vi "countrateJ&J.vi"() -> ()   [LabVIEW 2015]
uses:
  <vilib>/Platform/TimedLoop/XDataNode/timing_clust.ctl
  <vilib>/Platform/TimedLoop/XDataNode/nitl_modes.ctl
  <vilib>/Platform/TimedLoop/XDataNode/wakeup.ctl
  <vilib>/platform/TimedLoop/XDataNode/XDataNode.xnode
  <vilib>/Platform/TimedLoop/XDataNode/XDNodeRunTimeDep.lvlib
panel:
  out "Countrate":cluster{i32[], i32[]}(graph)
  out "output cluster":cluster{i32, dbl}
  in  "Controls":T1
  out "counts per Time Increment":dbl(knob) scale=0.0..100.0
  in  "stop":bool
  # "Demo count rate VI for Physics 434"
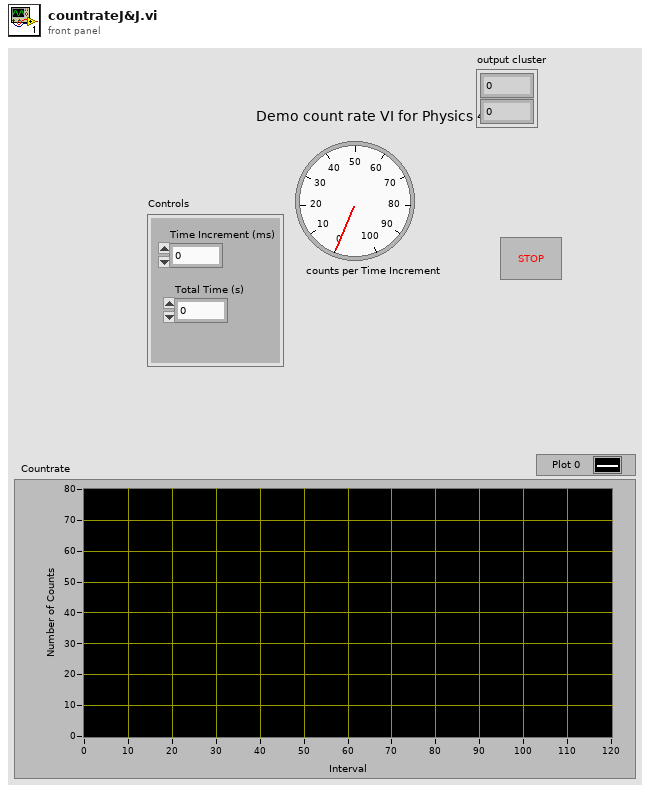
[diagram p1: front panel]
types:
  T1 = cluster{"Time Increment (ms)":i64, "Total Time (s)":dbl}
  T2 = enum16{"open", "replace", "create", "open or create", "replace or create", "replace or create with confirmation"}
  T3 = typedef "XDNodeRunTimeDep.lvlib/timing_clust.ctl" = cluster{"Expected End [f-1]":u64, "Actual End [f-1]":u64, "Finished Late? [f-1]":bool, "Expected End [i-1]":u64, "Actual End [i-1]":u64, "Finished Late? [i-1]":bool, "Expected Start [i]":u64, "Actual Start [i]":u64, "Expected Start [f]":u64, "Actual Start [f]":u64, "Source Name":string, "Structure Name":string, "Period":i64, "Deadline":i64, "Offset":i64, "Start":i64, "Priority":i32, "Timeout":i32, "Mode":T4, "Wakeup Reason":T5, "Error":errorcluster, "Source Type":string, "Secondary Source Type":string, "Global End Time":u64, "Global Start Time":u64, "Frame Duration":u64, "Iteration Duration":u64, "Assigned CPU":i32, "I/O Scan Engine Mode":u32}
  T4 = typedef "XDNodeRunTimeDep.lvlib/nitl_modes.ctl" = enum32{"No Change", "Process missed periods, maintain original phase", "Discard missed periods, maintain original phase", "Process missed periods, ignore original phase", "Discard missed periods, ignore original phase"}
  T5 = typedef "XDNodeRunTimeDep.lvlib/wakeup.ctl" = enum32{"Normal", "Aborted", "Asynchronous wakeup", "Timing source error", "Timed loop error", "Timeout"}
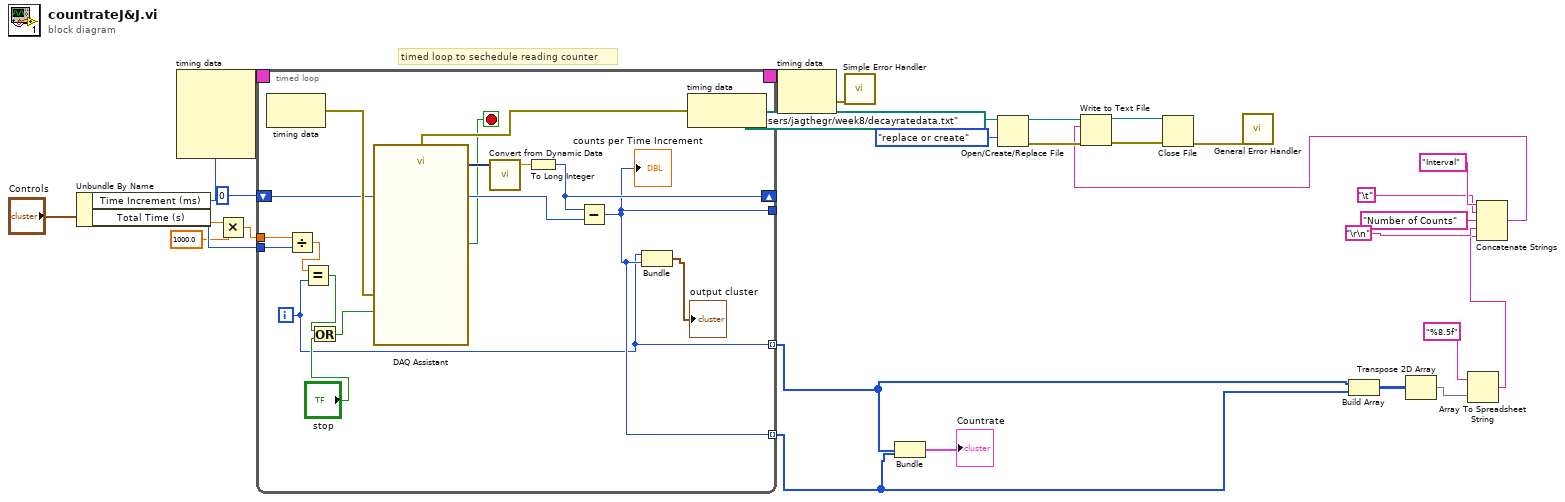
[diagram p0: block diagram]
diagram:
  # "timed loop to sechedule reading counter"
  n1 = Unbundle By Name("Controls") -> ("Time Increment (ms)"=w23:i64, "Total Time (s)"=w22:dbl)
  n2 = node-c288(w23) -> (w28:T3)  [unwired: 3 in]
  n3 = Multiply(x=w22, y=1000.0) -> (x*y=w20:dbl)
  n4 = timed-loop {
    timing: w28 -> [_]
    timing-out: [_] -> w27
    shift-right: [w43] -> _
    shift-left: 0 -> [w39]
    tunnel: [w30] -> _
    tunnel: w23 -> [w38]
    tunnel: w20 -> [w37]
    tunnel: [w30] -> w1 mode=indexing
    tunnel: [w29] -> w2 mode=indexing
    i -> [w29]
    stop <- w36 stop-if-true
    n5 = node-c288() -> (w40:errorcluster)  [unwired: 1 in]
    n6 = Divide(x=w37, y=w38) -> (x/y=w32:dbl)
    n7 = Equal?(x=w32, y=w29) -> (x = y?=w33:bool)
    n8 = Or(x=w33, y="stop") -> (x .or. y?=w34:bool)
    n9 = call "DAQ Assistant"("error in"=w40, "stop (F)"=w34) -> ("data"=w44:dynamicdata, "stopped"=w36:bool, "error out"=w41:errorcluster)  [unwired: 14 in, 1 out]
    n10 = call "Convert from Dynamic Data"("Dynamic Data Type"=w44) -> ("Scalar"=w42:dbl)  [unwired: 3 in]
    n11 = To Long Integer(number=w42) -> (32bit integer=w43:i32)
    n12 = Subtract(x=w43, y=w39) -> (x-y=w30:i32)
    "counts per Time Increment" <- w30
    n13 = Bundle(w29, w30) -> (→"output cluster":cluster{i32, i32})  [unwired: 1 in]
    n14 = node-c288(w41) -> ()  [unwired: 1 out]
  }
  n15 = node-c288(w27) -> (w25:errorcluster)
  n16 = call <vilib>:"Simple Error Handler.vi"("error in (no error)"=w25) -> ()  [unwired: 4 in, 5 out]
  n17 = Bundle(w2, w1) -> (→"Countrate":cluster{i32[], i32[]})  [unwired: 1 in]
  n18 = Open/Create/Replace File(file path (use dialog)=path "C:/Users/jagthegr/week8/decayratedata.txt", operation (0:open)=T2."replace or create") -> (refnum out=w15:refnum<file>, error out=w16:errorcluster)  [unwired: 4 in, 1 out]
  n19 = Build Array(w2, w1) -> (w3:i32[][])
  n20 = Transpose 2D Array(2D array=w3) -> (transposed array=w11:i32[][])
  n21 = Array To Spreadsheet String(array=w11, 3:"%8.5f" ("format string")) -> (spreadsheet string=w6:string)  [unwired: 1 in]
  n22 = Concatenate Strings("Interval" ("string"), "\t", "Number of Counts" ("string"), "\r\n", w6) -> (w5:string)
  n23 = Write to Text File(file (use dialog)=w15, text=w5, error in=w16) -> (refnum out=w14:refnum<file>, error out=w17:errorcluster)  [unwired: 1 in, 1 out]
  n24 = Close File(refnum=w14, error in=w17) -> (error out=w18:errorcluster)  [unwired: 1 out]
  n25 = call <vilib>:"General Error Handler.vi"("error in (no error)"=w18) -> ()  [unwired: 10 in, 5 out]
